vi "Process.vi"(8 "error in":errorcluster, 11 "UI_DSP_Config":refnum<class "UI_DSP_Config.lvclass">) -> (0 "error out":errorcluster, 3 "UI_DSP_Config out":refnum<class "UI_DSP_Config.lvclass">)   [LabVIEW 2016, in "UI_DSP_Config.lvclass"]
doc: "---------------------------------------------------------------\nJKI State Machine Objects™\nhttp://jki.net/state-machine-objects/\nCopyright (C) 2005-2015, JKI <info@jki.net>\nALL RIGHTS RESERVED"
uses:
  UI_DSP_Config.lvclass
  <vilib>/JKI/JKI SMO/SMO/SMO.lvclass
  <vilib>/JKI/JKI SMO/SMO/Typedefs/Parent Call--Enum.ctl
  DSP/DSP.lvclass
  DSP/Typedefs/LP_Config.ctl
  DSP.lockin/Typedefs/Lockin_Config.ctl
  DSP.lockin/DSP_lockin.lvclass
  <vilib>/Analysis/4window.llb/windowTd.ctl
  <vilib>/Analysis/NI_AALPro.lvlib
  <vilib>/measure/maspectr.llb/Power Spectrum and PSD Export Mode.ctl
  <vilib>/measure/NI_MAPro.lvlib
  DSP/Typedefs/FFT_Config.ctl
  DSP/Typedefs/PrivateEvents--DSP.RunCalculation.ctl
  C:/Program Files (x86)/National Instruments/LabVIEW 2016/vi.lib/JKI/JKI SMO/SMO/SMO.lvclass
  lockin/system.lvclass
  C:/user/patrick/hg/levy_inst_lockin.SMO/lvsrc/SMOs/instrument/instrument.lvclass
panel:
  in  "number of averages":u32 min=1
  in  "weighting mode":enum16{"Linear", "Exponential"}(ring)
  in  "averaging mode":T1(ring)
  in  "LP (Hz)":dbl
  in  "lockins config":T2(array[cluster])
  in  "power spectrum":bool
  in  "lockin":bool
  in  "LP prefilter":bool
  in  "60 Hz prefilter":bool
  in  "adjust offset":bool
  in  "adjust gain":bool
  in  "Close Window":bool
  # "For instructions on how to use the JKI State Machine Objects, examples and video tutorials, visit:\nhttp://jki.net/state-machine-objects/\n\nJKI State Machine Objects™\nhttp://jki.net/state-machine-objects/\nCopyright (C) 2005-2015, JKI <info@jki.net>\nALL RIGHTS RESERVED"
  # "This VIs should update DSP...when?\nOn any change? Live?"
  # "This VI should initialize by asking DSP\nwhat the current settings are...and populating\nthis controls."
  # "configDSP"
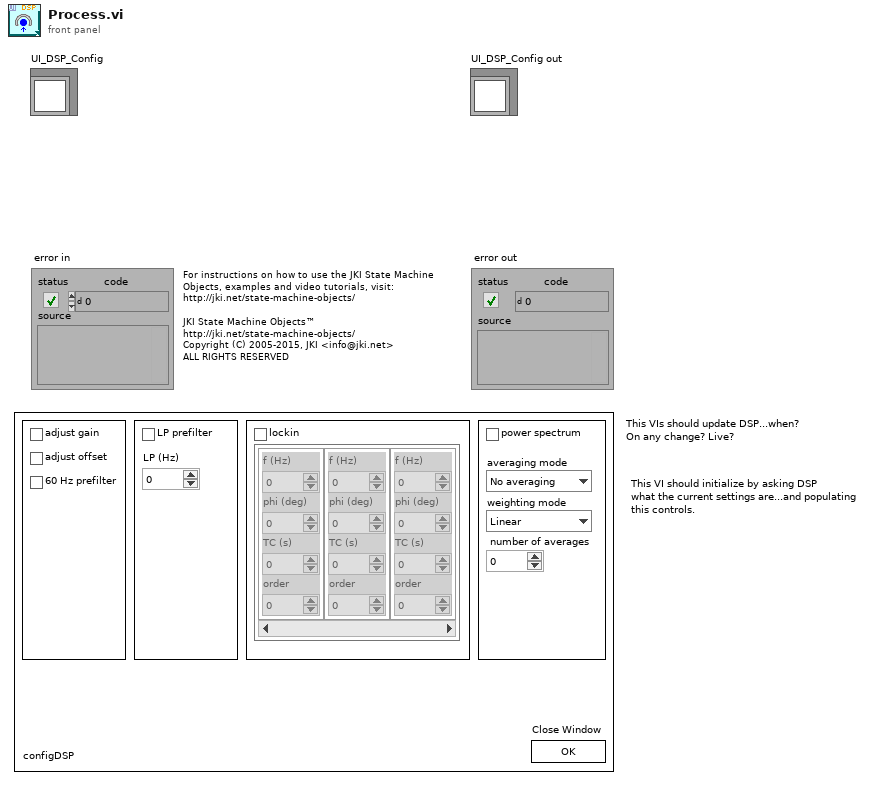
[diagram p1: front panel]
types:
  T1 = enum16{"No averaging", "Vector averaging", "RMS averaging", "Peak hold"}
  T2 = cluster{"f (Hz)":dbl, "phi (deg)":dbl, "TC (s)":dbl, "order":dbl}[]
  T3 = typedef "SMO.lvclass/Parent Call--Enum.ctl" = enum16{"Allows parent to run", "Does not request parent to run"}
  T4 = enum32{"invalid app kind", "Development System", "Run Time System", "Student Edition", "Embedded LabVIEW", "Evaluation", "Custom"}
  T5 = enum32{"Invalid", "Standard", "Closed", "Hidden", "Minimized", "Maximized"}
  T6 = enum32{"Bad", "Idle", "Run top level", "Running"}
  T7 = typedef "DSP.lvclass/PrivateEvents--DSP.RunCalculation.ctl" = cluster{"runCalculation":cluster{"adjust gain":bool, "subtract offset":bool, "60 Hz prefilter":bool, "LP prefilter":bool, "lockin":bool, "FFT":bool, "gain":dbl[], "offset":dbl[], "LP config":T8, "Lockin config":T9, "FFT config":T10}}
  T8 = typedef "DSP.lvclass/LP_Config.ctl" = cluster{"high cutoff freq [Hz]":dbl}
  T9 = typedef "DSP_lockin.lvclass/Lockin_Config.ctl" = cluster{" f (Hz)":dbl, "phi (deg)":dbl, "TC (s)":dbl, "order":i32}[]
  T10 = typedef "DSP.lvclass/FFT_Config.ctl" = cluster{"averaging parameters":cluster{"averaging mode":enum16{"No averaging", "Vector averaging", "RMS averaging", "Peak hold"}, "weighting mode":enum16{"Linear", "Exponential"}, "number of averages":u32}, "window":T11, "export mode":T12, "window parameter":dbl, "restart averaging (F)":bool}
  T11 = typedef "NI_AALPro.lvlib/windowTd.ctl" = u32
  T12 = typedef "NI_MAPro.lvlib/Power Spectrum and PSD Export Mode.ctl" = u16
  T13 = cluster{"Core":cluster{"Current VI Reference":refnum<vi>, "Close Panel on Exit?":bool, "error":errorcluster}, "Self Reference":refnum<class "UI_DSP_Config.lvclass">, "Your string data":string, "runCalculation":T7}
  T14 = cluster{"Current VI Reference":refnum<vi>, "Close Panel on Exit?":bool, "error":errorcluster}
  T15 = typedef "SMO.lvclass/Protected Events.ctl" = cluster{"StopProcesses":refnum<user-event>, "AbortProcesses":refnum<user-event>, "Config Changed":refnum<user-event>, "Dependency":refnum<user-event>}
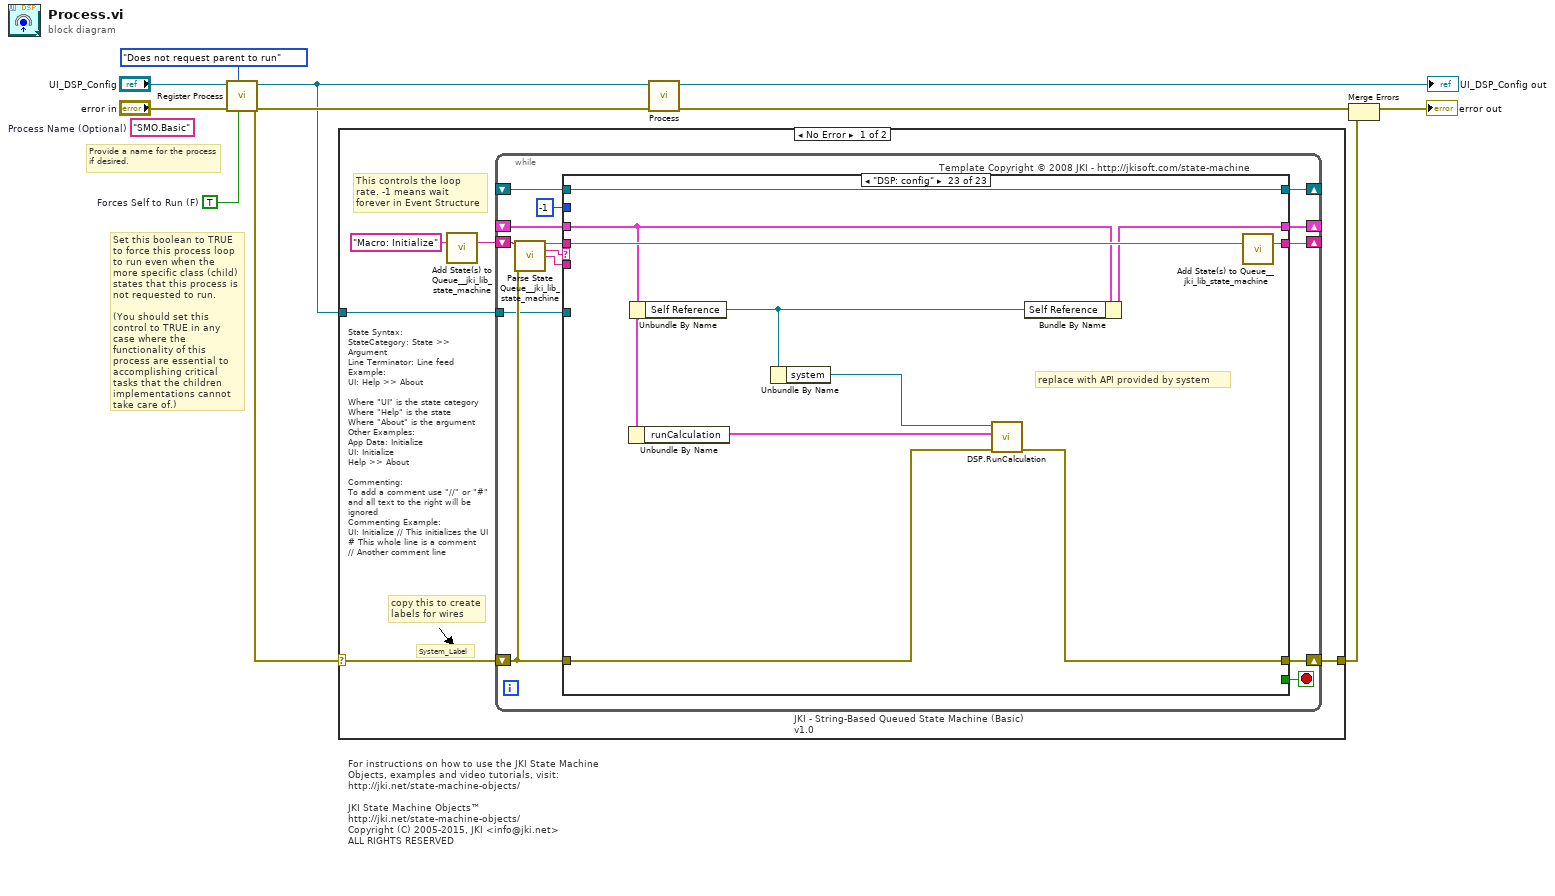
[diagram p0: block diagram]
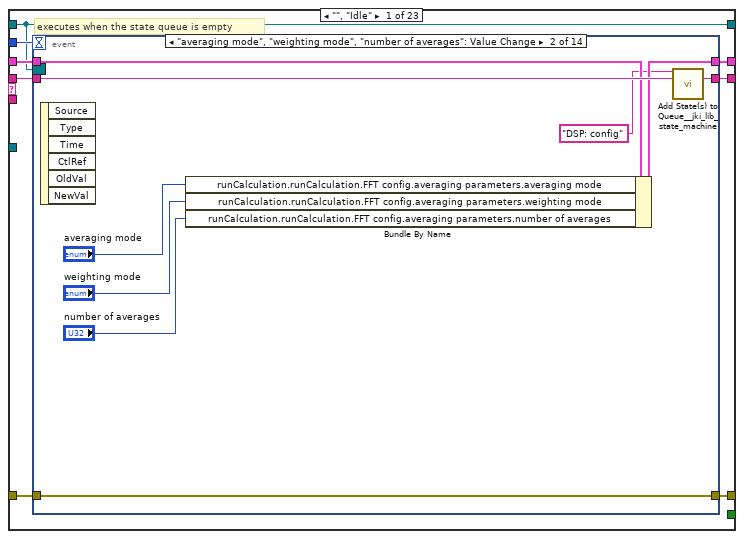
[diagram p2: hidden frame]
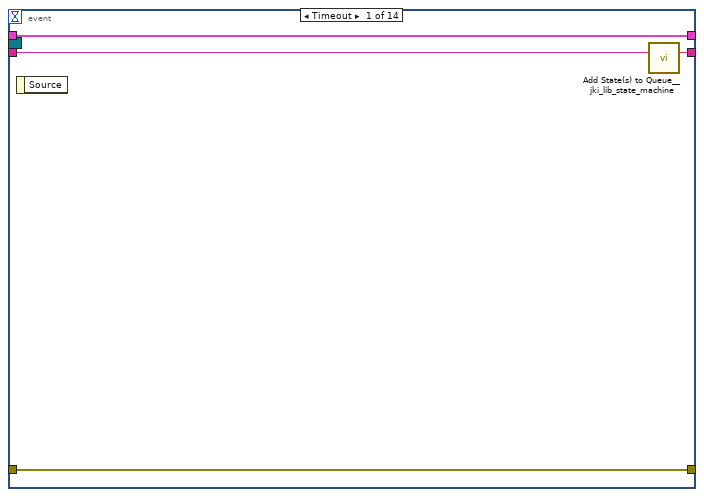
[diagram p3: hidden frame]
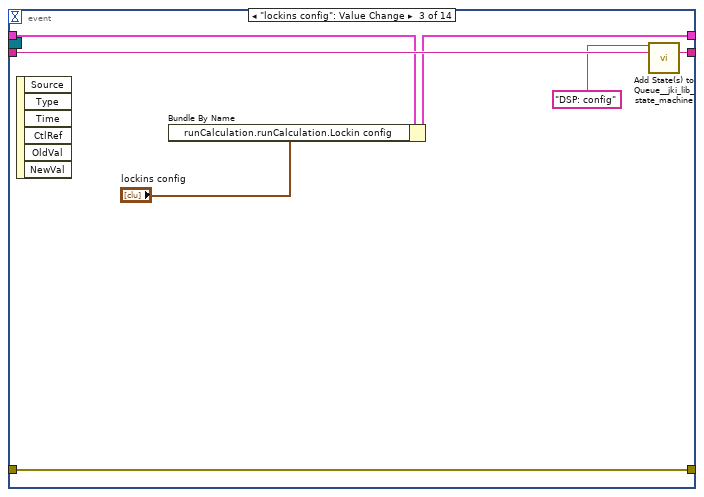
[diagram p4: hidden frame]
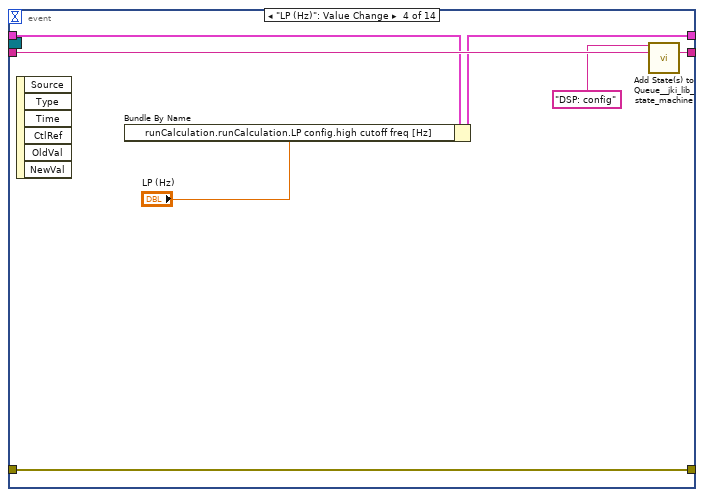
[diagram p5: hidden frame]
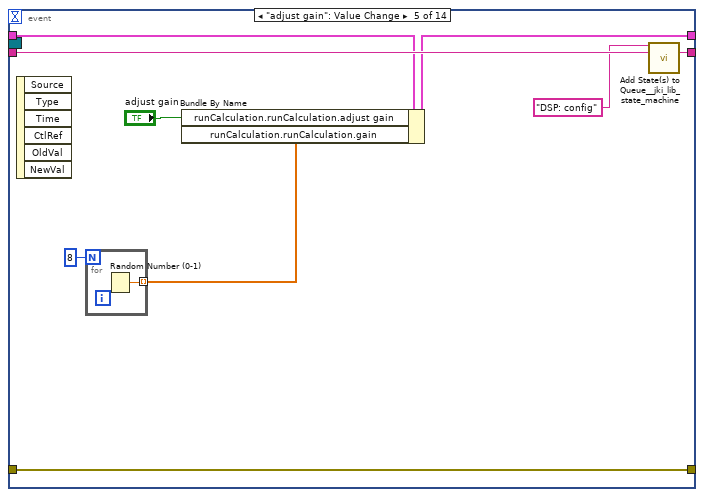
[diagram p6: hidden frame]
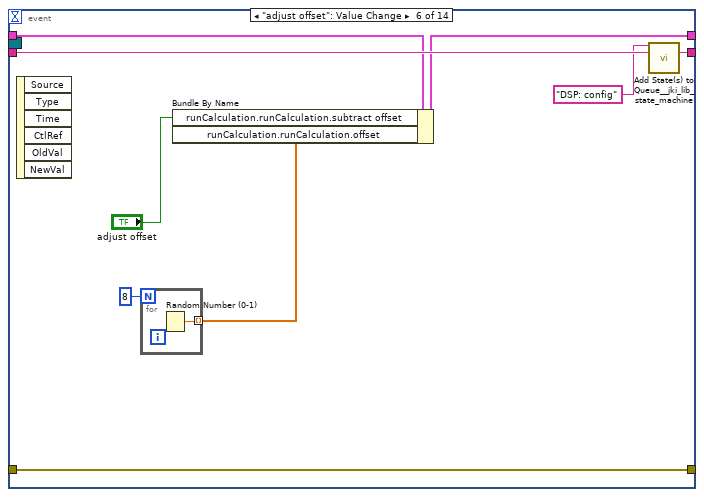
[diagram p7: hidden frame]
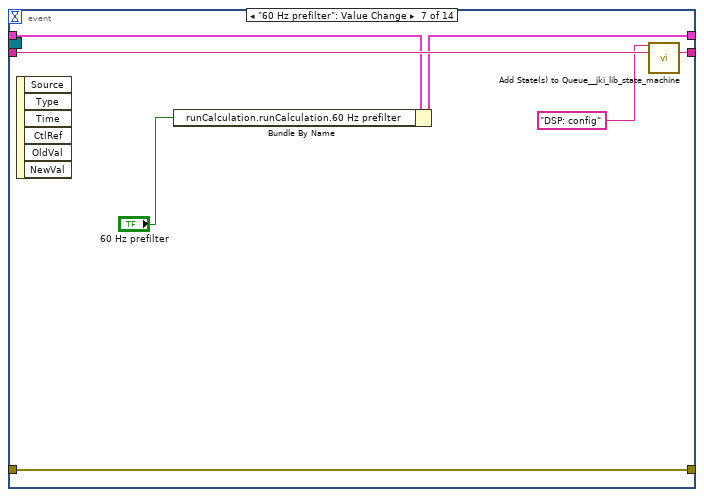
[diagram p8: hidden frame]
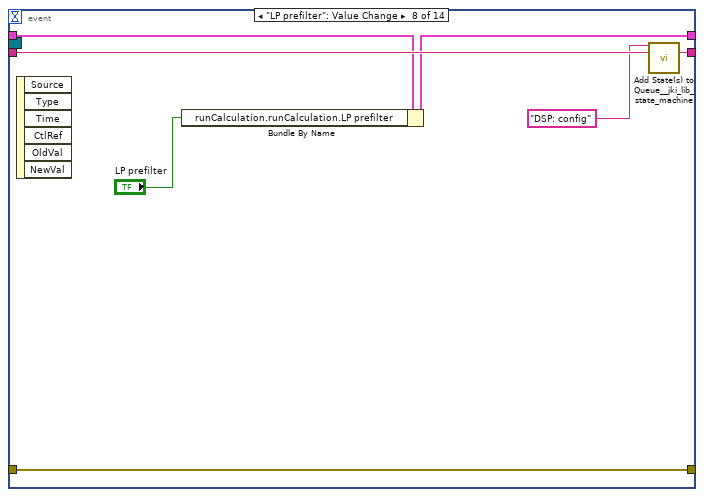
[diagram p9: hidden frame]
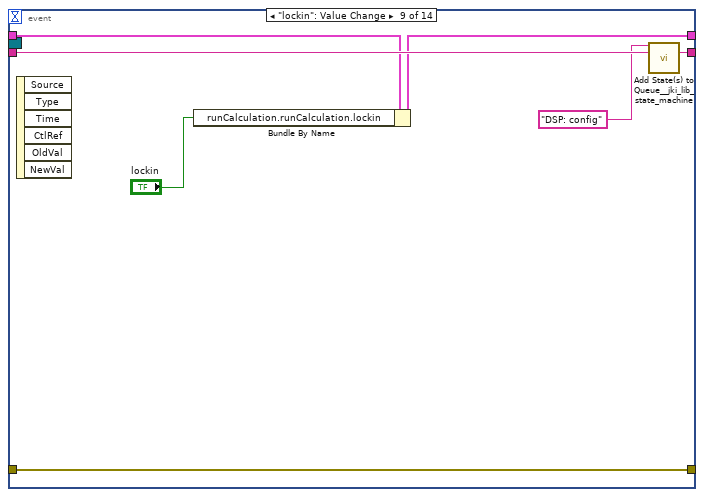
[diagram p10: hidden frame]
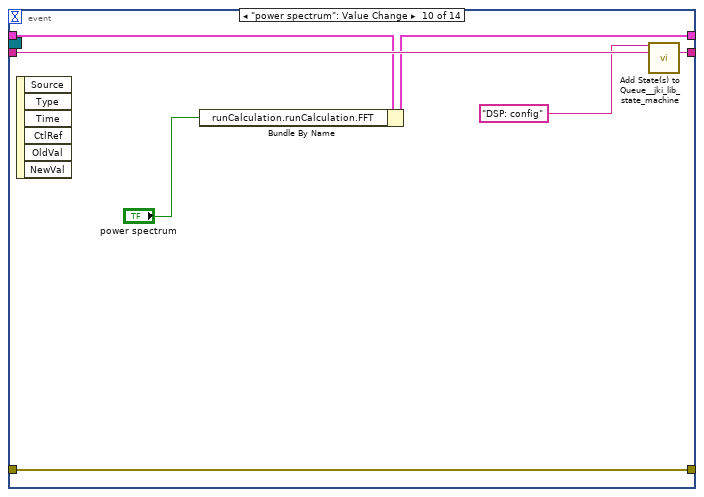
[diagram p11: hidden frame]
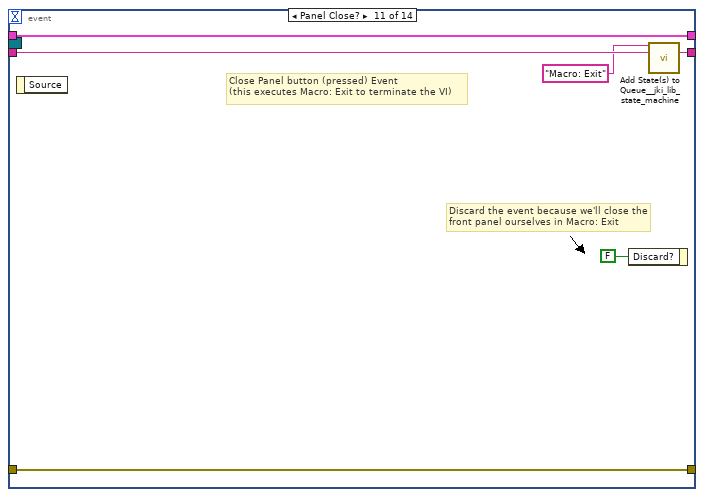
[diagram p12: hidden frame]
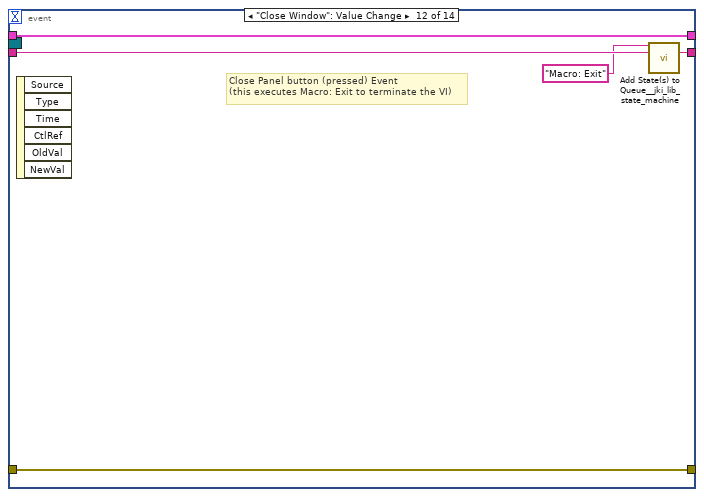
[diagram p13: hidden frame]
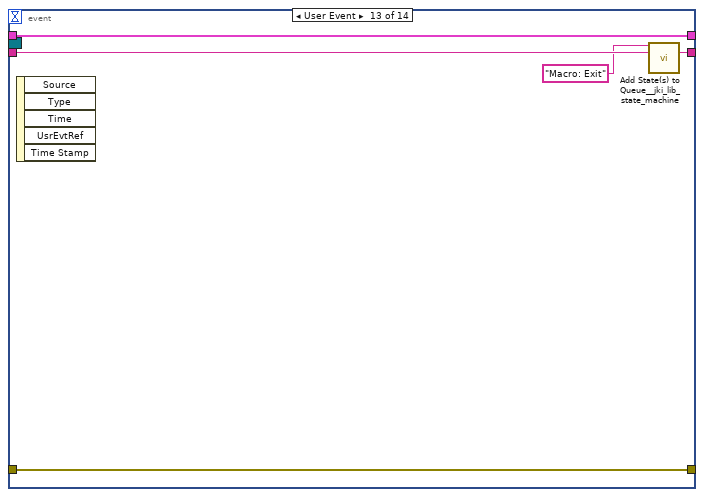
[diagram p14: hidden frame]
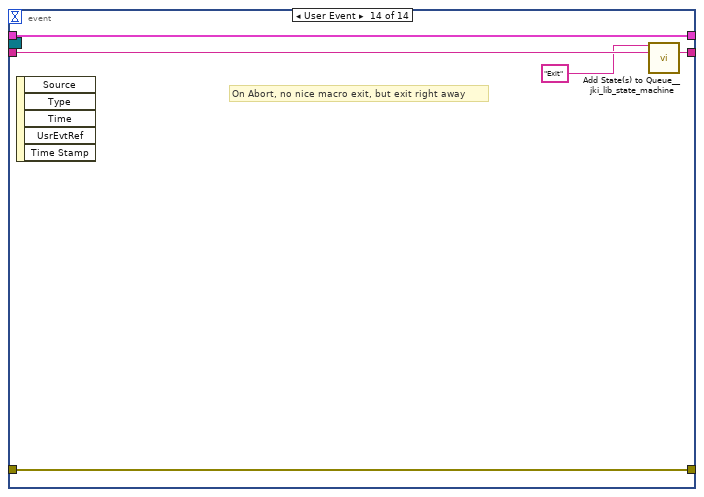
[diagram p15: hidden frame]
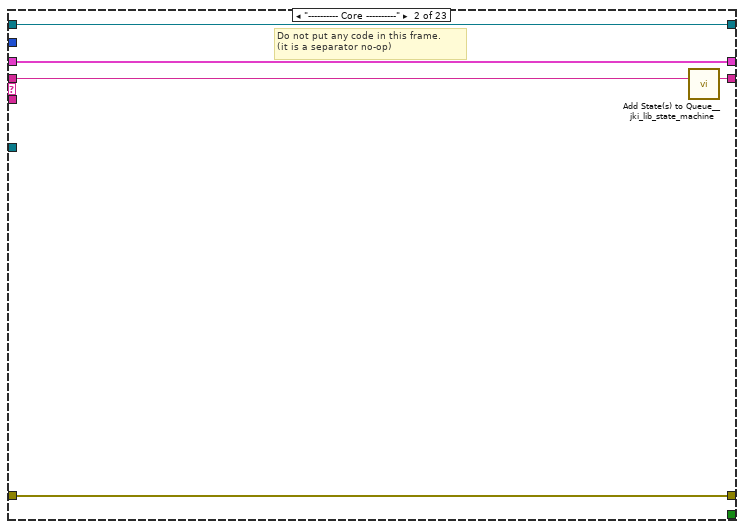
[diagram p16: hidden frame]
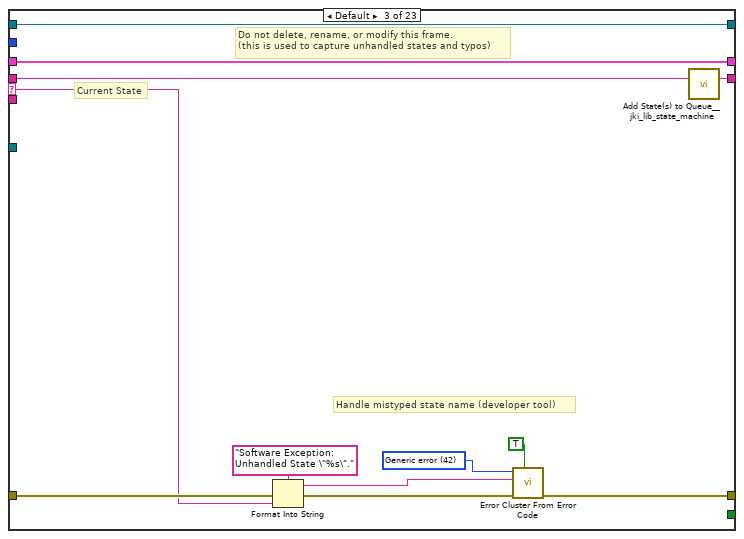
[diagram p17: hidden frame]
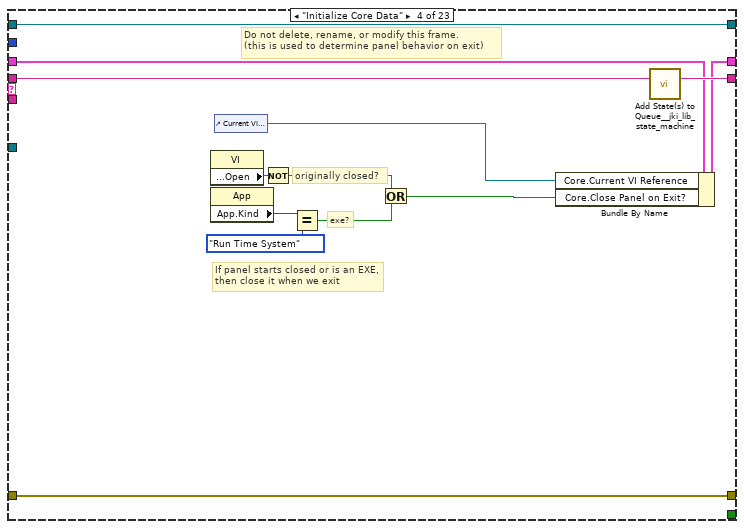
[diagram p18: hidden frame]
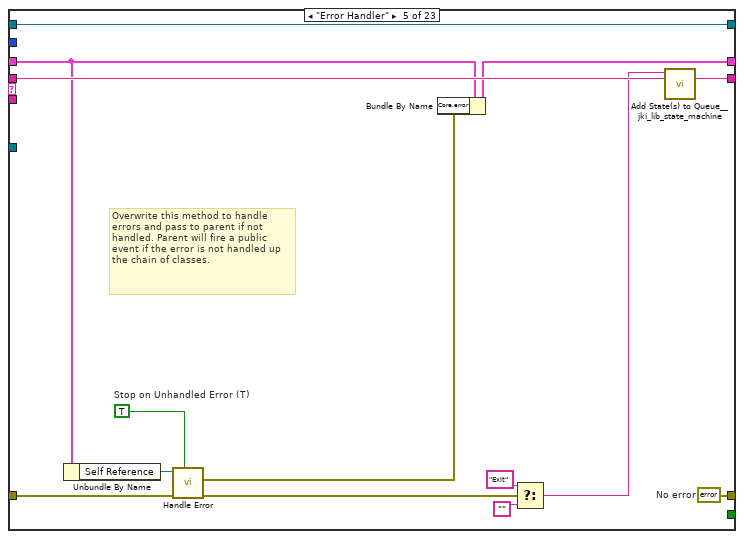
[diagram p19: hidden frame]
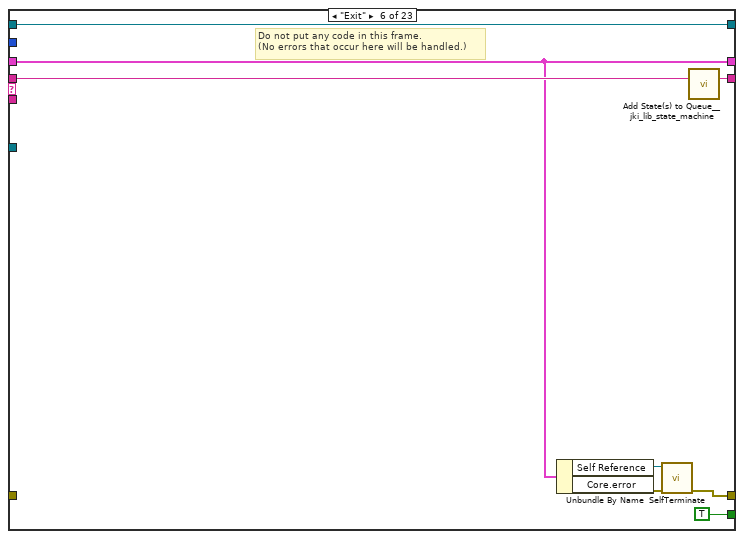
[diagram p20: hidden frame]
diagram:
  w1 = TRUE  # Forces Self to Run (F)
  (unwired) "SMO.Basic"  # Process Name (Optional)
  # "Provide a name for the process\nif desired."
  # "Set this boolean to TRUE to force this process loop to run even when the more specific class (child) states that this process is not requested to run.\n\n(You should set this control to TRUE in any case where the functionality of this process are essential to accomplishing critical tasks that the children implementations cannot take care of.)"
  # "For instructions on how to use the JKI State Machine Objects, examples and video tutorials, visit:\nhttp://jki.net/state-machine-objects/\n\nJKI State Machine Objects™\nhttp://jki.net/state-machine-objects/\nCopyright (C) 2005-2015, JKI <info@jki.net>\nALL RIGHTS RESERVED"
  n1 = call <vilib>:"Register Process.vi"("Forces Self to Run (F)"=w1, "Parent Call"=Parent_Call--Enum."Does not request parent to run", "error in (no error)"="error in", "SMO"="UI_DSP_Config") -> ("error out"=w7:errorcluster, "SMO out"=w6:refnum<class "UI_DSP_Config.lvclass">)  [unwired: 6 in]
  n2 = case shown="No Error" w7 {
    selector: w7 -> [w12 w356]
    tunnel: w6 -> [w13 _]
    tunnel: [w11 w356] -> w3
    frame No Error {
      # "State Syntax:\nStateCategory: State >> Argument\nLine Terminator: Line feed\nExample:\nUI: Help >> About\n\nWhere \"UI\" is the state category\nWhere \"Help\" is the state\nWhere \"About\" is the argument\nOther Examples:\nApp Data: Initialize\nUI: Initialize\nHelp >> About\n\nCommenting:\nTo add a comment use \"//\" or \"#\" and all text to the right will be ignored\nCommenting Example:\nUI: Initialize // This initializes the UI\n# This whole line is a comment\n// Another comment line"
      # "copy this to create labels for wires"
      # "This controls the loop rate. -1 means wait forever in Event Structure"
      # "System_Label"
      n3 = call <vilib>:"Add State(s) to Queue__jki_lib_state_machine.vi"("State(s) in (\"\")"="Macro: Initialize") -> ("States Out"=w15:string)  [unwired: 14 in]
      n4 = while "JKI - String-Based Queued State Machine (Basic) v1.0" {
        shift-right: [w22] -> _
        shift-left: _ -> [w21]
        shift-right: [w25] -> w11
        shift-left: w12 -> [w19]
        shift-right: [w24] -> _
        shift-left: w15 -> [w26]
        tunnel: w13 -> [w18]
        shift-right: [w17] -> _
        shift-left: _ -> [w16]
        stop <- w23 stop-if-true
        # "Template Copyright © 2008 JKI - http://jkisoft.com/state-machine"
        n5 = call <vilib>:"Parse State Queue__jki_lib_state_machine.vi"("State Queue"=w26, "Error In (no error)"=w19) -> ("Remaining States"=w28:string, "Current State"=w29:string, "Arguments"=w27:string)  [unwired: 11 in]
        n6 = case shown="\"DSP: config\"" w29 {
          selector: w29 -> [_ _ w140 _ _ _ _ _ _ _ _ _ _ _ _ _ _ _ _ _ _ _ _]
          tunnel: w28 -> [w37 w138 w144 w163 w177 w185 w190 w202 w209 w214 w220 w227 w243 w275 w289 w303 w308 w319 w324 w334 w340 w345 w355]
          tunnel: w27 -> [_ _ _ _ _ _ _ _ _ _ _ w221 w237 _ _ _ _ _ _ _ _ _ _]
          tunnel: w21 -> [w35 w135 w142 w154 w171 w179 w187 _ w204 w211 w218 w225 w239 w272 w285 w294 w305 w316 w321 w332 w338 w343 w349]
          tunnel: [w34 w136 w146 w160 w172 w178 w188 w197 w205 w212 w215 w222 w240 w273 w287 w301 w306 w310 w322 w327 w336 w341 w347] -> w25
          tunnel: w19 -> [w33 w136 w145 w160 w173 _ w188 w198 w206 w212 w216 w223 w241 w273 w287 w301 w306 w311 w322 w328 w336 w341 w346]
          tunnel: [w36 w137 w143 w162 w176 w184 w189 w201 w208 w213 w219 w226 w242 w274 w288 w302 w307 w318 w323 w333 w339 w344 w354] -> w24
          tunnel: [_ _ _ _ _ TRUE _ _ _ _ _ _ _ _ _ _ _ _ _ _ _ _ _] -> w23
          tunnel: [w32 w135 w142 w161 w170 w179 w187 w200 w204 w211 w218 w225 w239 w272 w285 w294 w305 w316 w321 w332 w338 w343 w352] -> w22
          tunnel: -1 ("Timeout") -> [w31 _ _ _ _ _ _ _ _ _ _ _ _ _ _ _ _ _ _ _ _ _ _]
          tunnel: w18 -> [_ _ _ _ _ _ _ w195 _ _ _ _ _ _ _ _ _ _ _ _ _ _ _]
          tunnel: [w30 w134 w139 w151 w175 w182 w186 w193 w203 w210 w217 w224 w236 w271 w286 w295 w304 w317 w320 w331 w337 w342 w353] -> w17
          tunnel: w16 -> [w30 w134 w139 w151 w175 w182 w186 w193 w203 w210 w217 w224 w236 w271 w286 w295 w304 w317 w320 _ w337 w342 w353]
          frame "", "Idle" {
            # "executes when the state queue is empty"
            n7 = event shown="[1] \"averaging mode\", \"weighting mode\", \"number of averages\": Value Change" {
              selector: w30 -> [_ _ _ _ _ _ _ _ _ _ _ _ _ _]
              dyn-events: _ -> [_ _ _ _ _ _ _ _ _ _ _ _ _ _]
              timeout: w31 -> [_ _ _ _ _ _ _ _ _ _ _ _ _ _]
              tunnel: w37 -> [w41 w50 w57 w64 w73 w83 w91 w98 w105 w112 w118 w123 w128 w133]
              tunnel: [w40 w49 w56 w63 w72 w82 w90 w97 w104 w111 w117 w122 w127 w132] -> w36
              tunnel: w35 -> [w39 w47 w54 w61 w70 w80 w88 w95 w102 w109 w115 w120 w125 w130]
              tunnel: [w38 w48 w55 w62 w71 w81 w89 w96 w103 w110 w116 w121 w126 w131] -> w34
              tunnel: w33 -> [w38 w48 w55 w62 w71 w81 w89 w96 w103 w110 w116 w121 w126 w131]
              tunnel: [w39 w46 w53 w60 w69 w79 w87 w94 w101 w108 w115 w120 w125 w130] -> w32
              event Timeout {
                n8 = event-data() -> ()  [unwired: 1 in, 1 out]
                n9 = call <vilib>:"Add State(s) to Queue__jki_lib_state_machine.vi"("State(s) in (\"\")"=w41) -> ("States Out"=w40:string)  [unwired: 14 in]
              }
              event "averaging mode", "weighting mode", "number of averages": Value Change {
                n10 = event-data() -> ()  [unwired: 1 in, 6 out]
                n11 = Bundle By Name(cluster=w47, "runCalculation.runCalculation.FFT config.averaging parameters.averaging mode"="averaging mode", "runCalculation.runCalculation.FFT config.averaging parameters.weighting mode"="weighting mode", "runCalculation.runCalculation.FFT config.averaging parameters.number of averages"="number of averages") -> (w46:T13)
                n12 = call <vilib>:"Add State(s) to Queue__jki_lib_state_machine.vi"("State(s) in Front (\"\")"="DSP: config" ("State(s) in Front (\"\")"), "State(s) in (\"\")"=w50) -> ("States Out"=w49:string)  [unwired: 13 in]
              }
              event "lockins config": Value Change {
                n13 = event-data() -> ()  [unwired: 1 in, 6 out]
                n14 = Bundle By Name(cluster=w54, "runCalculation.runCalculation.Lockin config"="lockins config") -> (w53:T13)
                n15 = call <vilib>:"Add State(s) to Queue__jki_lib_state_machine.vi"("State(s) in Front (\"\")"="DSP: config" ("State(s) in Front (\"\")"), "State(s) in (\"\")"=w57) -> ("States Out"=w56:string)  [unwired: 13 in]
              }
              event "LP (Hz)": Value Change {
                n16 = event-data() -> ()  [unwired: 1 in, 6 out]
                n17 = Bundle By Name(cluster=w61, "runCalculation.runCalculation.LP config.high cutoff freq [Hz]"="LP (Hz)") -> (w60:T13)
                n18 = call <vilib>:"Add State(s) to Queue__jki_lib_state_machine.vi"("State(s) in Front (\"\")"="DSP: config" ("State(s) in Front (\"\")"), "State(s) in (\"\")"=w64) -> ("States Out"=w63:string)  [unwired: 13 in]
              }
              event "adjust gain": Value Change {
                n19 = event-data() -> ()  [unwired: 1 in, 6 out]
                n20 = for {
                  N: 8 -> [_]
                  tunnel: [w74] -> w65 mode=indexing
                  n21 = Random Number (0-1)() -> (number: 0 to 1=w74:dbl)
                }
                n22 = Bundle By Name(cluster=w70, "runCalculation.runCalculation.adjust gain"="adjust gain", "runCalculation.runCalculation.gain"=w65) -> (w69:T13)
                n23 = call <vilib>:"Add State(s) to Queue__jki_lib_state_machine.vi"("State(s) in Front (\"\")"="DSP: config" ("State(s) in Front (\"\")"), "State(s) in (\"\")"=w73) -> ("States Out"=w72:string)  [unwired: 13 in]
              }
              event "adjust offset": Value Change {
                n24 = event-data() -> ()  [unwired: 1 in, 6 out]
                n25 = for {
                  N: 8 -> [_]
                  tunnel: [w84] -> w75 mode=indexing
                  n26 = Random Number (0-1)() -> (number: 0 to 1=w84:dbl)
                }
                n27 = Bundle By Name(cluster=w80, "runCalculation.runCalculation.subtract offset"="adjust offset", "runCalculation.runCalculation.offset"=w75) -> (w79:T13)
                n28 = call <vilib>:"Add State(s) to Queue__jki_lib_state_machine.vi"("State(s) in Front (\"\")"="DSP: config" ("State(s) in Front (\"\")"), "State(s) in (\"\")"=w83) -> ("States Out"=w82:string)  [unwired: 13 in]
              }
              event "60 Hz prefilter": Value Change {
                n29 = event-data() -> ()  [unwired: 1 in, 6 out]
                n30 = Bundle By Name(cluster=w88, "runCalculation.runCalculation.60 Hz prefilter"="60 Hz prefilter") -> (w87:T13)
                n31 = call <vilib>:"Add State(s) to Queue__jki_lib_state_machine.vi"("State(s) in Front (\"\")"="DSP: config" ("State(s) in Front (\"\")"), "State(s) in (\"\")"=w91) -> ("States Out"=w90:string)  [unwired: 13 in]
              }
              event "LP prefilter": Value Change {
                n32 = event-data() -> ()  [unwired: 1 in, 6 out]
                n33 = Bundle By Name(cluster=w95, "runCalculation.runCalculation.LP prefilter"="LP prefilter") -> (w94:T13)
                n34 = call <vilib>:"Add State(s) to Queue__jki_lib_state_machine.vi"("State(s) in Front (\"\")"="DSP: config" ("State(s) in Front (\"\")"), "State(s) in (\"\")"=w98) -> ("States Out"=w97:string)  [unwired: 13 in]
              }
              event "lockin": Value Change {
                n35 = event-data() -> ()  [unwired: 1 in, 6 out]
                n36 = Bundle By Name(cluster=w102, "runCalculation.runCalculation.lockin"="lockin") -> (w101:T13)
                n37 = call <vilib>:"Add State(s) to Queue__jki_lib_state_machine.vi"("State(s) in Front (\"\")"="DSP: config" ("State(s) in Front (\"\")"), "State(s) in (\"\")"=w105) -> ("States Out"=w104:string)  [unwired: 13 in]
              }
              event "power spectrum": Value Change {
                n38 = event-data() -> ()  [unwired: 1 in, 6 out]
                n39 = Bundle By Name(cluster=w109, "runCalculation.runCalculation.FFT"="power spectrum") -> (w108:T13)
                n40 = call <vilib>:"Add State(s) to Queue__jki_lib_state_machine.vi"("State(s) in Front (\"\")"="DSP: config" ("State(s) in Front (\"\")"), "State(s) in (\"\")"=w112) -> ("States Out"=w111:string)  [unwired: 13 in]
              }
              event Panel Close? {
                # "Discard the event because we'll close the front panel ourselves in Macro: Exit"
                # "Close Panel button (pressed) Event\n(this executes Macro: Exit to terminate the VI)"
                n41 = event-data() -> ()  [unwired: 1 in, 1 out]
                n42 = event-data("Discard?"=FALSE) -> ()  [unwired: 1 in, 1 out]
                n43 = call <vilib>:"Add State(s) to Queue__jki_lib_state_machine.vi"("State(s) in Front (\"\")"="Macro: Exit", "State(s) in (\"\")"=w118) -> ("States Out"=w117:string)  [unwired: 13 in]
              }
              event "Close Window": Value Change {
                # "Close Panel button (pressed) Event\n(this executes Macro: Exit to terminate the VI)"
                n44 = event-data() -> ()  [unwired: 1 in, 6 out]
                n45 = call <vilib>:"Add State(s) to Queue__jki_lib_state_machine.vi"("State(s) in Front (\"\")"="Macro: Exit", "State(s) in (\"\")"=w123) -> ("States Out"=w122:string)  [unwired: 13 in]
              }
              event User Event {
                n46 = event-data() -> ()  [unwired: 1 in, 5 out]
                n47 = call <vilib>:"Add State(s) to Queue__jki_lib_state_machine.vi"("State(s) in Front (\"\")"="Macro: Exit", "State(s) in (\"\")"=w128) -> ("States Out"=w127:string)  [unwired: 13 in]
              }
              event User Event {
                # "On Abort, no nice macro exit, but exit right away"
                n48 = event-data() -> ()  [unwired: 1 in, 5 out]
                n49 = call <vilib>:"Add State(s) to Queue__jki_lib_state_machine.vi"("State(s) in Front (\"\")"="Exit", "State(s) in (\"\")"=w133) -> ("States Out"=w132:string)  [unwired: 13 in]
              }
            }
          }
          frame "---------- Core ----------" {
            # "Do not put any code in this frame.\n(it is a separator no-op)"
            n50 = call <vilib>:"Add State(s) to Queue__jki_lib_state_machine.vi"("State(s) in (\"\")"=w138) -> ("States Out"=w137:string)  [unwired: 14 in]
          }
          frame Default {
            w149 = 42 items=["No error", "Argument error", "Memory is full", "Out of zone", "End of file", "File already open", "Generic file I/O error", "File not found", "File permission error", "Disk is full", "Duplicate path", "Too many files open", "System feature not enabled", "Resource file not found", "Cannot add resource", "Resource not found", "Image not found", "Image memory error", "Pen does not exist", "Config type invalid", "Config token not found", "Config parse error", "Config memory error", "Bad external code format", "Bad external code offset", "External code not present", "Null window", "Destroy window error", "Null menu", "Print aborted", "Bad print record", "Print driver error", "Windows error during printing", "Memory error during printing", "Print dialog error", "Generic print error", "Invalid device refnum", "Device not found", "Device parameter error", "Device unit error", "Cannot open device", "Device call aborted", "Generic error", "Cancelled by user", "Object ID too low", "Object ID too high", "Object not in heap", "Unknown heap", "Unknown object (invalid DefProc)", "Unknown object (DefProc not in table)", "Message out of range", "Invalid (null) method", "Unknown message", "Manager call not supported", "Bad address", "Network operation in progress", "Network operation timed out", "Connection is busy", "Network attribute not supported", "Network error", "Address in use", "System out of memory", "Connection aborted", "Connection refused", "Not connected", "Already connected", "Connection closed", "Initialization error (interapplication manager)", "Bad occurrence", "Wait on unbound occurrence handler", "Occurrence queue overflow", "Datalog type conflict", "Unused", "Unrecognized type (interapplication manager)", "Memory corrupt", "Failed to make temporary DLL", "Old CIN version", "Drag socket not found", "Failed to load drop-object", "Failed to register OLE object", "Failed to release OLE object", "Format specifier type mismatch", "Unknown format specifier", "Too few format specifiers", "Too many format specifiers", "Scan failed", "Newer CIN version", "Error converting to variant", "Runtime menu error", "Password tampered", "Variant attribute not found", "Incompatible variant data type", "Event data is not available", "Event Store is not present", "Occurrence is not found", "Event Queue is not created", "Event info is not available", "Refnum passed is NULL", "Error retrieving Class GUID", "Error retrieving CoClass GUID", "Error retrieving TypeLib GUID.", "Bad built application magic bytes.", "Specific driver is different from the specific driver associated with the Logical Name.", "There is no session opened to the class driver.", "Max Error", "MAX - Error with config objects", "MAX - Error loading configuration", "MAX - Group not supported"]
            # "Current State"
            # "Do not delete, rename, or modify this frame.\n(this is used to capture unhandled states and typos)"
            # "Handle mistyped state name (developer tool)"
            n51 = Format Into String(format string="Software Exception: Unhandled State \"%s\"." ("message"), error in=w145, w140) -> (resulting string=w148:string, error out=w147:errorcluster)  [unwired: 1 in]
            n52 = call <vilib>:"Error Cluster From Error Code.vi"("show call chain? (False)"=TRUE, "error in (no error)"=w147, "error message (\"\")"=w148, "error code (0)"=w149) -> ("error out"=w146:errorcluster)  [unwired: 5 in]
            n53 = call <vilib>:"Add State(s) to Queue__jki_lib_state_machine.vi"("State(s) in (\"\")"=w144) -> ("States Out"=w143:string)  [unwired: 14 in]
          }
          frame "Initialize Core Data" {
            # "Do not delete, rename, or modify this frame.\n(this is used to determine panel behavior on exit)"
            # "originally closed?"
            # "exe?"
            # "If panel starts closed or is an EXE, then close it when we exit"
            n54 = property class="VI"() -> ("Front Panel.Open"=w159:bool)  [unwired: 2 in, 2 out]
            n55 = property class="App"() -> ("App.Kind"=w158:T4)  [unwired: 2 in, 2 out]
            n56 = control-ref of="Current VI Reference"() -> (w152:refnum<vi>)
            n57 = Not(x=w159) -> (.not. x?=w156:bool)
            n58 = Equal?(x=w158, y=T4."Run Time System" ("Application:Kind")) -> (x = y?=w155:bool)
            n59 = Or(x=w156, y=w155) -> (x .or. y?=w153:bool)
            n60 = Bundle By Name(cluster=w154, "Core.Current VI Reference"=w152, "Core.Close Panel on Exit?"=w153) -> (w161:T13)
            n61 = call <vilib>:"Add State(s) to Queue__jki_lib_state_machine.vi"("State(s) in (\"\")"=w163) -> ("States Out"=w162:string)  [unwired: 14 in]
          }
          frame "Error Handler" {
            w164 = TRUE  # Stop on Unhandled Error (T)
            w172 = errorcluster {"status"=FALSE, "code"=0, "source"=""}  # No error
            # "Overwrite this method to handle errors and pass to parent if not handled. Parent will fire a public event if the error is not handled up the chain of classes."
            n62 = Unbundle By Name(w171) -> ("Self Reference"=w174:refnum<class "UI_DSP_Config.lvclass">)
            n63 = call-dynamic "Handle Error.vi"("Stop on Unhandled Error (T)"=w164, "error in"=w173, "SMO"=w174) -> ("handling error"=w165:errorcluster, "Unhandled error"=w168:errorcluster)  [unwired: 6 in, 1 out]
            n64 = Bundle By Name(cluster=w171, "Core.error"=w168) -> (w170:T13)
            n65 = Select(t="Exit", s=w165, f="") -> (s? t:f=w169:string)
            n66 = call <vilib>:"Add State(s) to Queue__jki_lib_state_machine.vi"("State(s) in Front (\"\")"=w169, "State(s) in (\"\")"=w177) -> ("States Out"=w176:string)  [unwired: 13 in]
          }
          frame "Exit" {
            # "Do not put any code in this frame.\n(No errors that occur here will be handled.)"
            n67 = Unbundle By Name(w179) -> ("Self Reference"=w180:refnum<class "UI_DSP_Config.lvclass">, "Core.error"=w181:errorcluster)
            n68 = call <vilib>:"SelfTerminate.vi"("error in (no error)"=w181, "SMO in"=w180) -> ("error out"=w178:errorcluster)  [unwired: 8 in, 1 out]
            n69 = call <vilib>:"Add State(s) to Queue__jki_lib_state_machine.vi"("State(s) in (\"\")"=w185) -> ("States Out"=w184:string)  [unwired: 14 in]
          }
          frame "---------- Data ----------" {
            # "Do not put any code in this frame.\n(It is a separator no-op. You can make a copy of this frame to create a new Data frame)"
            n70 = call <vilib>:"Add State(s) to Queue__jki_lib_state_machine.vi"("State(s) in (\"\")"=w190) -> ("States Out"=w189:string)  [unwired: 14 in]
          }
          frame "Data: Initialize" {
            w191 = T7 {"runCalculation"={"adjust gain"=FALSE, "subtract offset"=FALSE, "60 Hz prefilter"=FALSE, "LP prefilter"=FALSE, "lockin"=FALSE, "FFT"=FALSE, "gain"=[], "offset"=[], "LP config"={"high cutoff freq [Hz]"=0.0}, "Lockin config"=[], "FFT config"={"averaging parameters"={"averaging mode"=enum."No averaging", "weighting mode"=enum."Linear", "number of averages"=0}, "window"=0, "export mode"=0, "window parameter"=0.0, "restart averaging (F)"=FALSE}}}  # runCalculation
            w192 = T14 {"Current VI Reference"=refnum, "Close Panel on Exit?"=FALSE, "error"={"status"=FALSE, "code"=0, "source"=""}}  # Core
            w196 = refnum<class "UI_DSP_Config.lvclass"> refnum  # Self Reference
            w199 = ""  # Your string data
            # "do not delete - used by framework"
            # "Expand Bundle to add new data elements to shift register data."
            # "Add new data here."
            # "Data names and types of shift register data are defined by this bundle."
            # "Initialize the shift-register data, here.\n(data names are defined by what you wire into the bundle function)"
            n71 = Variant To Data(error in=w198, type=w196, Variant=w195) -> (data=w194:refnum<class "UI_DSP_Config.lvclass">, error out=w197:errorcluster)
            n72 = Bundle("Core"=w192, "Self Reference"=w194, "Your string data"=w199, "runCalculation"=w191) -> (w200:T13)  [unwired: 1 in]
            n73 = call <vilib>:"Add State(s) to Queue__jki_lib_state_machine.vi"("State(s) in (\"\")"=w202) -> ("States Out"=w201:string)  [unwired: 14 in]
          }
          frame "Data: Cleanup" {
            # "Cleanup any data and references, here.\n(this is called automatically, by the Macro: Exit)"
            n74 = Unbundle By Name(w204) -> ("Core.Current VI Reference"=w207:refnum<vi>)
            n75 = Close Reference(reference=w207, error in (no error)=w206) -> (error out=w205:errorcluster)
            n76 = call <vilib>:"Add State(s) to Queue__jki_lib_state_machine.vi"("State(s) in (\"\")"=w209) -> ("States Out"=w208:string)  [unwired: 14 in]
          }
          frame "---------- UI ----------" {
            # "Do not put any code in this frame.\n(It is a separator no-op. You can make a copy of this frame to create a new UI frame)"
            n77 = call <vilib>:"Add State(s) to Queue__jki_lib_state_machine.vi"("State(s) in (\"\")"=w214) -> ("States Out"=w213:string)  [unwired: 14 in]
          }
          frame "UI: Initialize" {
            # "Initialize the User Interface, here.\n(this is called automatically, by the Macro: Init)"
            n78 = call <userlib>:"Fit VI window to Largest Dec__ogtk.vi"("error in (no error)"=w216) -> ("error out"=w215:errorcluster)  [unwired: 5 in, 1 out]
            n79 = call <vilib>:"Add State(s) to Queue__jki_lib_state_machine.vi"("State(s) in (\"\")"=w220) -> ("States Out"=w219:string)  [unwired: 14 in]
          }
          frame "UI: Cursor Set" {
            # "Argument"
            # "Initialize the User Interface, here.\n(this is called automatically, by the Macro: Init)"
            n80 = disable-structure shown="Default" {
              disable-tunnel: w223 -> [w228 w231]
              disable-tunnel: [w228 w230] -> w222
              disable-tunnel: w221 -> [_ w229]
              frame condition #0 {
              }
              frame condition #1 (active) {
                n81 = case shown="\"Idle\", Default" w229 {
                  tunnel: w231 -> [w233 w235]
                  tunnel: [w232 w234] -> w230
                  frame "Idle", Default {
                    n82 = call <vilib>:"Unset Busy.vi"("error in (no error)"=w233) -> ("error out"=w232:errorcluster)  [unwired: 10 in]
                  }
                  frame "Busy" {
                    n83 = call <vilib>:"Set Busy.vi"("error in (no error)"=w235) -> ("error out"=w234:errorcluster)  [unwired: 9 in, 1 out]
                  }
                }
              }
            }
            n84 = call <vilib>:"Add State(s) to Queue__jki_lib_state_machine.vi"("State(s) in (\"\")"=w227) -> ("States Out"=w226:string)  [unwired: 14 in]
          }
          frame "UI: Front Panel State" {
            # "Argument"
            # "Set Front Panel Open or Closed\n(Usage: \"UI: Front Panel State >> Open|Close\")"
            n85 = Unbundle By Name(w239) -> ("Core.Current VI Reference"=w238:refnum<vi>)
            n86 = disable-structure shown="Default" {
              disable-tunnel: w241 -> [w247 w270]
              disable-tunnel: [w246 w270] -> w240
              disable-tunnel: w238 -> [w245 _]
              disable-tunnel: w237 -> [w244 _]
              frame condition #0 (active) {
                n87 = case shown="\"Close\"" w244 {
                  tunnel: w247 -> [w251 w264]
                  tunnel: [w253 w265] -> w246
                  tunnel: w245 -> [w252 w262]
                  frame "Open", Default {
                    n88 = property class="VI"(reference=w252, error in=w251) -> (reference out=w249:refnum<vi>, error out=w250:errorcluster, "FP.State"=w248:T5)
                    n89 = case shown="\"Closed\"" w248 {
                      tunnel: [w256 w259] -> w253
                      tunnel: w250 -> [w255 w259]
                      tunnel: w249 -> [w254 _]
                      frame "Closed" {
                        n90 = invoke class="VI" method="FP.Open"(reference=w254, error in=w255, "Activate"=TRUE, "State"=T5."Standard") -> (error out=w256:errorcluster)  [unwired: 1 in, 4 out]
                      }
                      frame Default {
                      }
                    }
                  }
                  frame "Close" {
                    n91 = property class="VI"(reference=w262, error in=w264) -> (reference out=w261:refnum<vi>, error out=w263:errorcluster, "FP.State"=w260:T5)
                    n92 = case shown="Default" w260 {
                      tunnel: [w266 w269] -> w265
                      tunnel: w263 -> [w266 w268]
                      tunnel: w261 -> [_ w267]
                      frame "Invalid", "Closed" {
                      }
                      frame Default {
                        n93 = invoke class="VI" method="FP.Close"(reference=w267, error in=w268) -> (error out=w269:errorcluster)  [unwired: 1 in, 2 out]
                      }
                    }
                  }
                }
              }
              frame condition #1 {
              }
            }
            n94 = call <vilib>:"Add State(s) to Queue__jki_lib_state_machine.vi"("State(s) in (\"\")"=w243) -> ("States Out"=w242:string)  [unwired: 14 in]
          }
          frame "---------- Macro ----------" {
            # "Do not put any code in this frame.\n(It is a separator no-op. You can make a copy of this frame to create a new Macro frame)"
            n95 = call <vilib>:"Add State(s) to Queue__jki_lib_state_machine.vi"("State(s) in (\"\")"=w275) -> ("States Out"=w274:string)  [unwired: 14 in]
          }
          frame "Macro: Initialize" {
            w280 = "UI: Initialize\nUI: Front Panel State >> Open"  # UI: Initialize UI: Front Panel State >> Open
            w276 = "Process: Sync"
            # "Initialization Macro\n(This is called once, when the VI starts)"
            n96 = control-ref of="This VI"() -> (w278:refnum<vi>)
            n97 = property class="VI"(reference=w278) -> ("Exec.State"=w277:T6)  [unwired: 1 in, 2 out]
            n98 = Equal?(x=w277, y=T6."Run top level") -> (x = y?=w283:bool)
            n99 = Select(t=w276, s=w283, f="") -> ()  [unwired: 1 out]
            n100 = call <vilib>:"Add State(s) to Queue__jki_lib_state_machine.vi"("State(s) in Front (\"\")"="Data: Initialize\nInitialize Core Data\nEvents: Register", "State(s) in (\"\")"=w276, "State(s) at Back (\"\")"=w280) -> ("States Out"=w279:string)  [unwired: 12 in]
            n101 = call <vilib>:"Add State(s) to Queue__jki_lib_state_machine.vi"("State(s) in Front (\"\")"=w279, "State(s) in (\"\")"=w289) -> ("States Out"=w288:string)  [unwired: 13 in]
          }
          frame "Macro: Exit" {
            # "Exit Macro\n(This is called once, when the VI exits)"
            n102 = Unbundle By Name(w294) -> ("Core.Close Panel on Exit?"=w300:bool)
            n103 = Select(t="UI: Front Panel State >> Close", s=w300, f="") -> (s? t:f=w297:string)
            n104 = call <vilib>:"Add State(s) to Queue__jki_lib_state_machine.vi"("State(s) in Front (\"\")"="Data: Cleanup\nEvents: Unregister", "State(s) in (\"\")"="Process: Sync", "State(s) at Back (\"\")"="Exit") -> ("States Out"=w291:string)  [unwired: 12 in]
            n105 = call <vilib>:"Add State(s) to Queue__jki_lib_state_machine.vi"("State(s) in (\"\")"=w297, "State(s) at Back (\"\")"=w291) -> ("States Out"=w296:string)  [unwired: 13 in]
            n106 = call <vilib>:"Add State(s) to Queue__jki_lib_state_machine.vi"("State(s) in Front (\"\")"=w296, "State(s) in (\"\")"=w303) -> ("States Out"=w302:string)  [unwired: 13 in]
          }
          frame "---------- Process ----------" {
            # "Template Separator\n(You can make a copy of, or modify, this frame)"
            n107 = call <vilib>:"Add State(s) to Queue__jki_lib_state_machine.vi"("State(s) in (\"\")"=w308) -> ("States Out"=w307:string)  [unwired: 14 in]
          }
          frame "Process: Sync" {
            n108 = Unbundle By Name(w316) -> ("Self Reference"=w312:refnum<class "UI_DSP_Config.lvclass">)
            n109 = call <vilib>:"WaitOnProcessSync.vi"("error in (no error)"=w311, "SMO"=w312) -> ("error out"=w310:errorcluster, "Don't run?"=w315:bool)  [unwired: 7 in, 1 out]
            n110 = Select(t="Data: Cleanup\nEvents: Unregister\nExit", s=w315, f="") -> (s? t:f=w309:string)
            n111 = call <vilib>:"Add State(s) to Queue__jki_lib_state_machine.vi"("State(s) in Front (\"\")"=w309, "State(s) in (\"\")"=w319) -> ("States Out"=w318:string)  [unwired: 13 in]
          }
          frame "---------- Events ----------" {
            # "Template Separator\n(You can make a copy of, or modify, this frame)"
            n112 = call <vilib>:"Add State(s) to Queue__jki_lib_state_machine.vi"("State(s) in (\"\")"=w324) -> ("States Out"=w323:string)  [unwired: 14 in]
          }
          frame "Events: Register" {
            # "Expand to add\nmore events"
            n113 = Unbundle By Name(w332) -> ("Self Reference"=w329:refnum<class "UI_DSP_Config.lvclass">)
            n114 = call <vilib>:"GetProtectedEvents.vi"("SMO"=w329) -> ("error out"=w325:errorcluster, "SMO Protected Events"=w330:T15)  [unwired: 8 in, 1 out]
            n115 = register-events(w330) -> (reference out=w331:refnum<event-registration>, error out=w326:errorcluster)  [unwired: 2 in]
            n116 = Merge Errors(w328, w326, w325) -> (w327:errorcluster)
            n117 = call <vilib>:"Add State(s) to Queue__jki_lib_state_machine.vi"("State(s) in (\"\")"=w334) -> ("States Out"=w333:string)  [unwired: 14 in]
          }
          frame "Events: Unregister" {
            n118 = Unregister For Events(event registration refnum=w337, error in=w336) -> (error out=w335:errorcluster)
            n119 = call <vilib>:"Clear Errors.vi"("error in (no error)"=w335) -> ()  [unwired: 5 in, 2 out]
            n120 = call <vilib>:"Add State(s) to Queue__jki_lib_state_machine.vi"("State(s) in (\"\")"=w340) -> ("States Out"=w339:string)  [unwired: 14 in]
          }
          frame "---------- Action ----------" {
            n121 = call <vilib>:"Add State(s) to Queue__jki_lib_state_machine.vi"("State(s) in (\"\")"=w345) -> ("States Out"=w344:string)  [unwired: 14 in]
          }
          frame "DSP: config" {
            # "replace with API provided by system"
            n122 = Unbundle By Name(w349) -> ("runCalculation"=w348:T7)
            n123 = Unbundle By Name(w349) -> ("Self Reference"=w351:refnum<class "UI_DSP_Config.lvclass">)
            n124 = Unbundle By Name(w351) -> ("system"=w350:refnum<class "system.lvclass">)
            n125 = call "DSP.RunCalculation.vi"("error in (no error)"=w346, "runCalculation"=w348, "DSP"=w350) -> ("error out"=w347:errorcluster)  [unwired: 7 in, 1 out]
            n126 = Bundle By Name(cluster=w349, "Self Reference"=w351) -> (w352:T13)
            n127 = call <vilib>:"Add State(s) to Queue__jki_lib_state_machine.vi"("State(s) in (\"\")"=w355) -> ("States Out"=w354:string)  [unwired: 14 in]
          }
        }
      }
    }
    frame Error {
    }
  }
  n128 = call-parent "Process.vi"("error in"=w7, "SMO"=w6) -> ("error out"=w4:errorcluster, "SMO out"=→"UI_DSP_Config out":refnum<class "UI_DSP_Config.lvclass">)  [unwired: 8 in]
  n129 = Merge Errors(w4, w3) -> (→"error out":errorcluster)
